vi "Test.vi"(11 "试验项目":T1(ring)) -> ()   [LabVIEW 2012]
uses:
  resultShow.vi
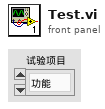
[diagram p1: front panel]
types:
  T1 = enum32{"功能", "输入输出特性", "电流特性", "传感器特性", "空载", "逆向空载", "振动", "7", "8", "9", "10", "11", "12", "13"}
  T2 = enum16{"selectdata", "selectsave", "selectlist", "selectshow"}
  T3 = cluster{"max":dbl, "min":dbl, "uripp":dbl, "average":dbl}
  T4 = cluster{"vaule":dbl, "vaule":dbl, "limitL":dbl, "limitH":dbl}
  T5 = typedef "svc_Spectrum Info.ctl" = cluster{"channel name":string, "description":string, "x-axis units":T6, "spectral info":cluster{"spectrum type":T7, "linear/dB":enum16{"linear", "dB"}, "window":u16, "window size":i32, "FFT size":i32}, "engineering units":T8, "custom label":string, "dB reference [EU]":dbl, "peak units":enum16{"rms", "peak", "peak-peak"}, "weighting filter":T9, "spectral density?":bool, "unit label":string, "spectrum skewed?":bool, "complimentary spectrum units":T10}
  T6 = typedef "svc_X-Axis Units.ctl" = u16
  T7 = typedef "svc_Spectrum Type.ctl" = enum16{"FFT Spectrum [complex]", "Amplitude [Magnitude]", "Power [Magnitude^2]", "Cross Spectrum [complex]", "Frequency Response [Complex]"}
  T8 = typedef "svc_Engineering Units Text Ring.ctl" = u16
  T9 = typedef "svc_Weighting Filter Text Ring.ctl" = u16
  T10 = typedef "svc_Complimentary Spectrum Units.ctl" = enum16{"none", "radians", "degrees", "cycles", "imaginary"}
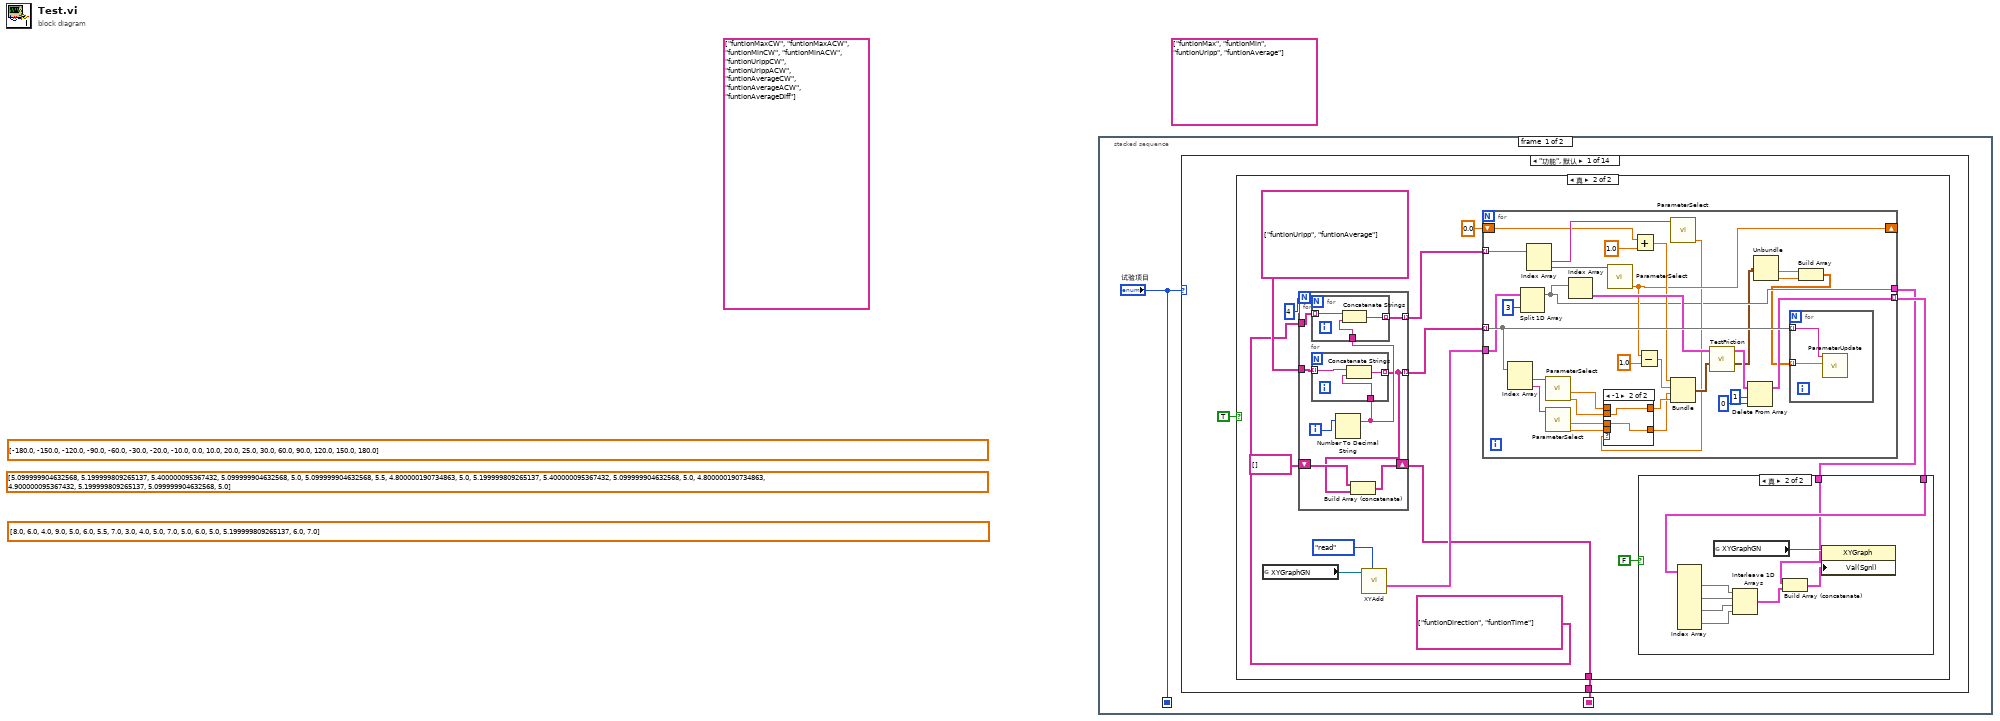
[diagram p0: block diagram]
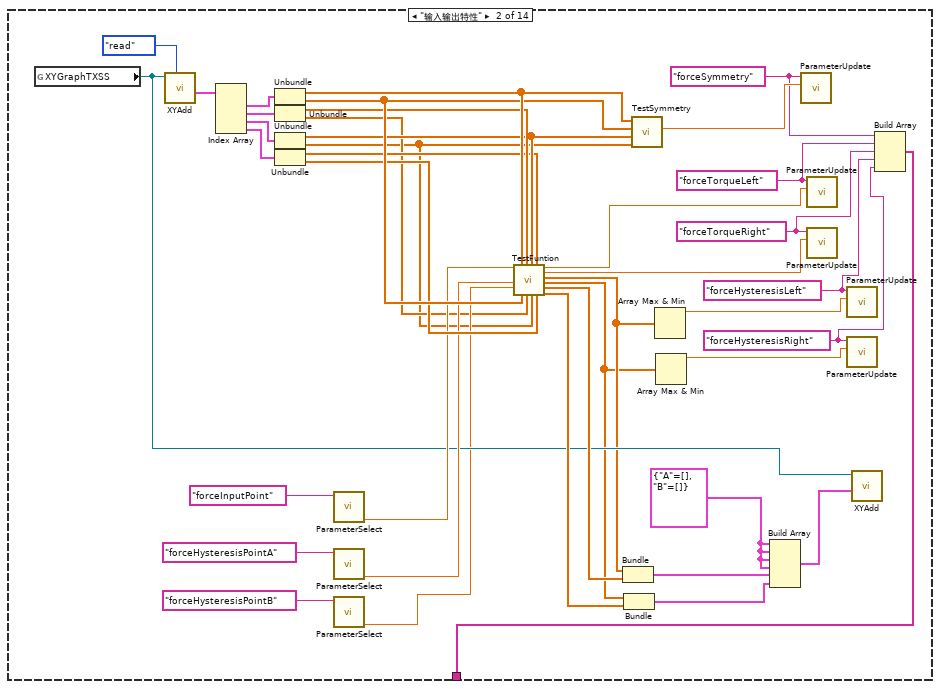
[diagram p5: hidden frame]
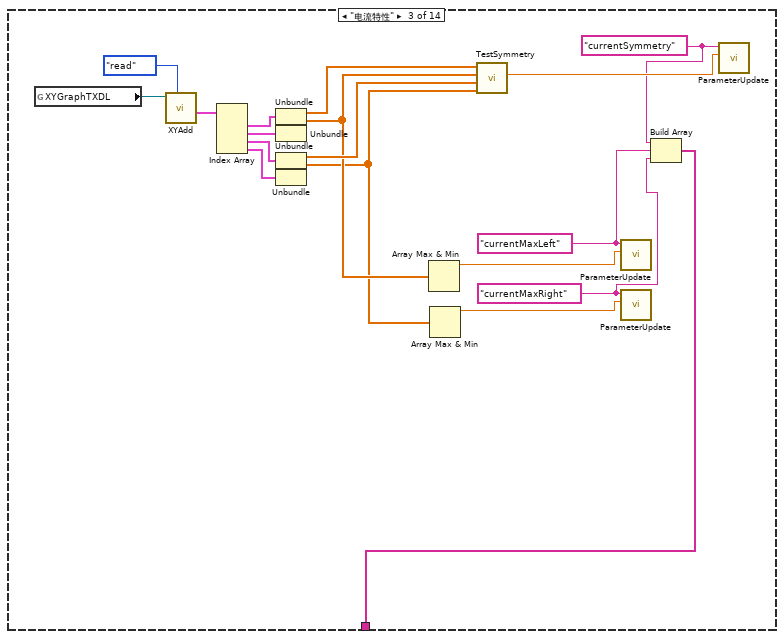
[diagram p6: hidden frame]
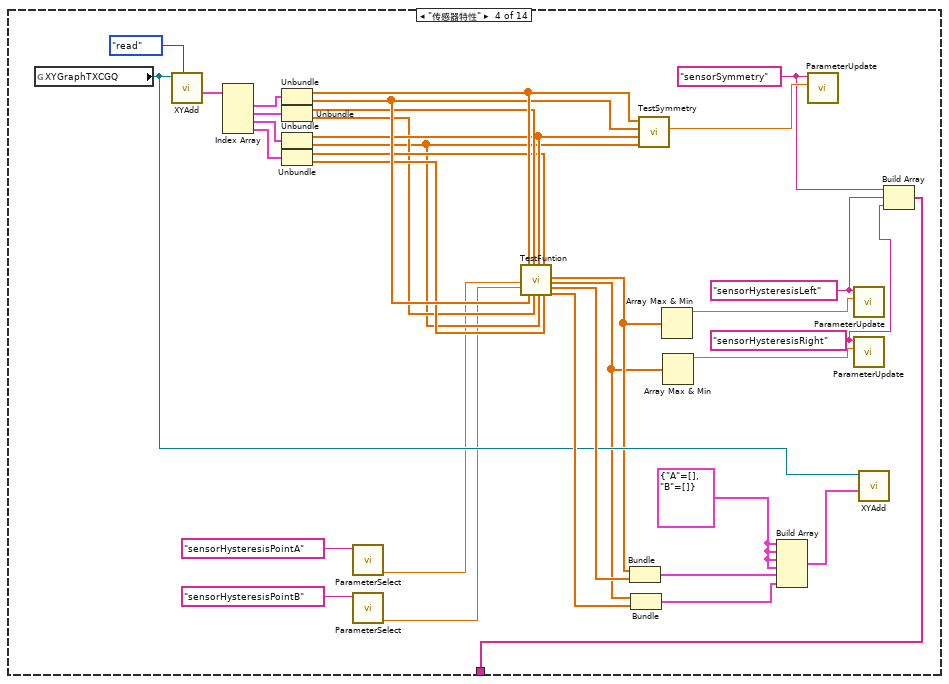
[diagram p7: hidden frame]
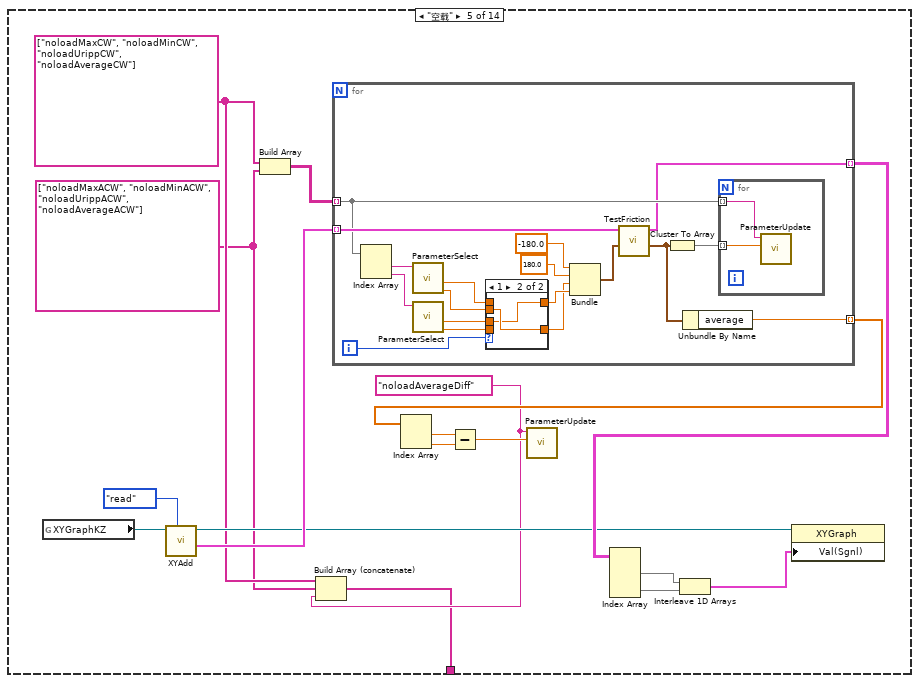
[diagram p8: hidden frame]
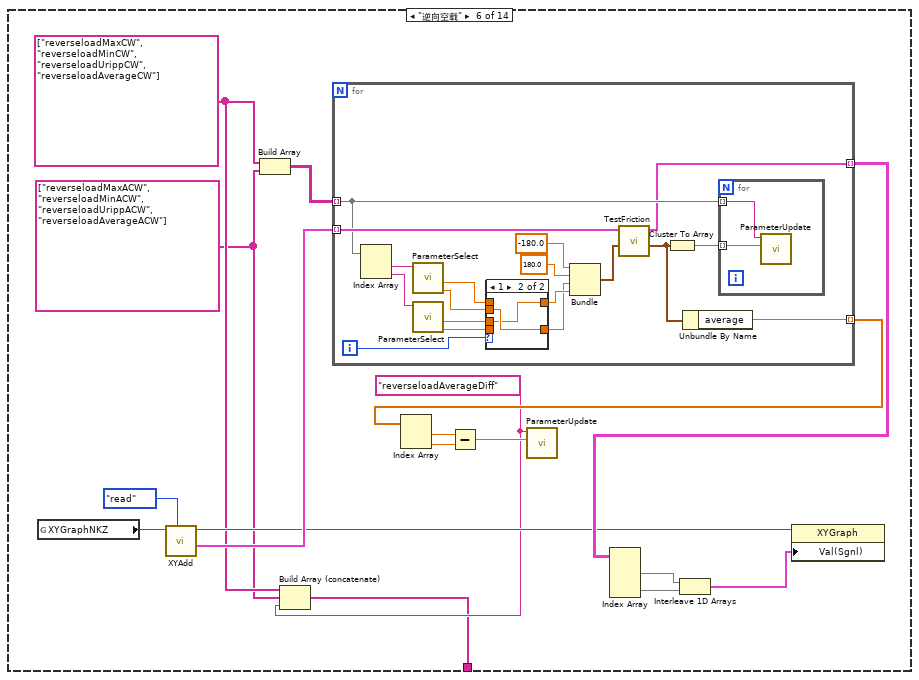
[diagram p10: hidden frame]
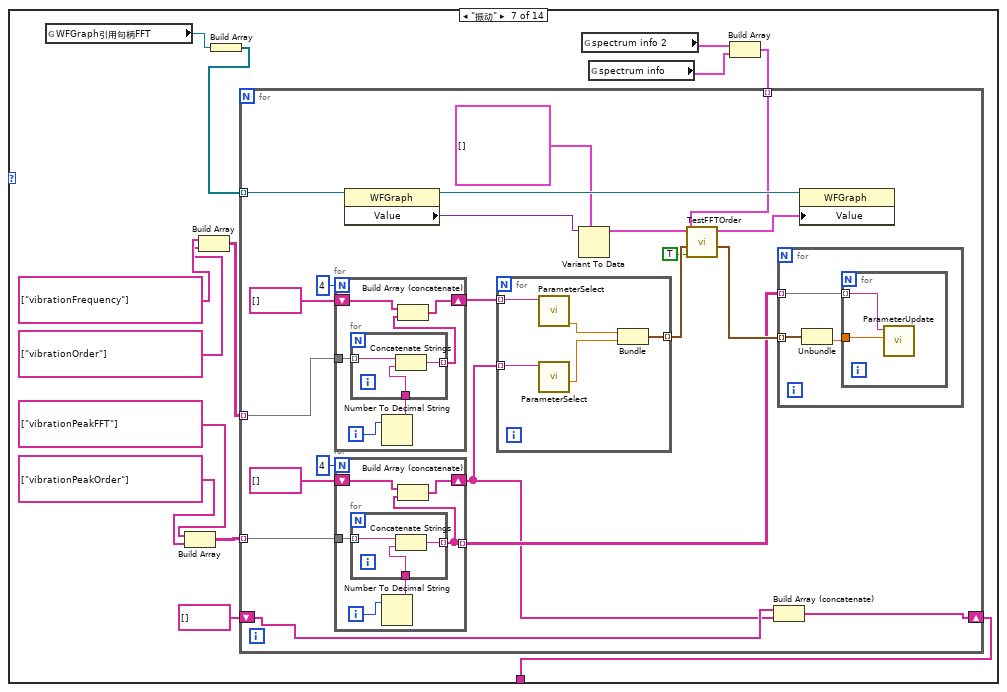
[diagram p12: hidden frame]
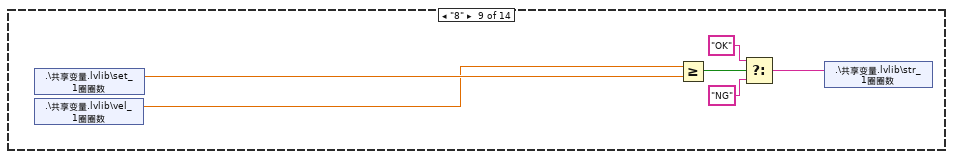
[diagram p14: hidden frame]
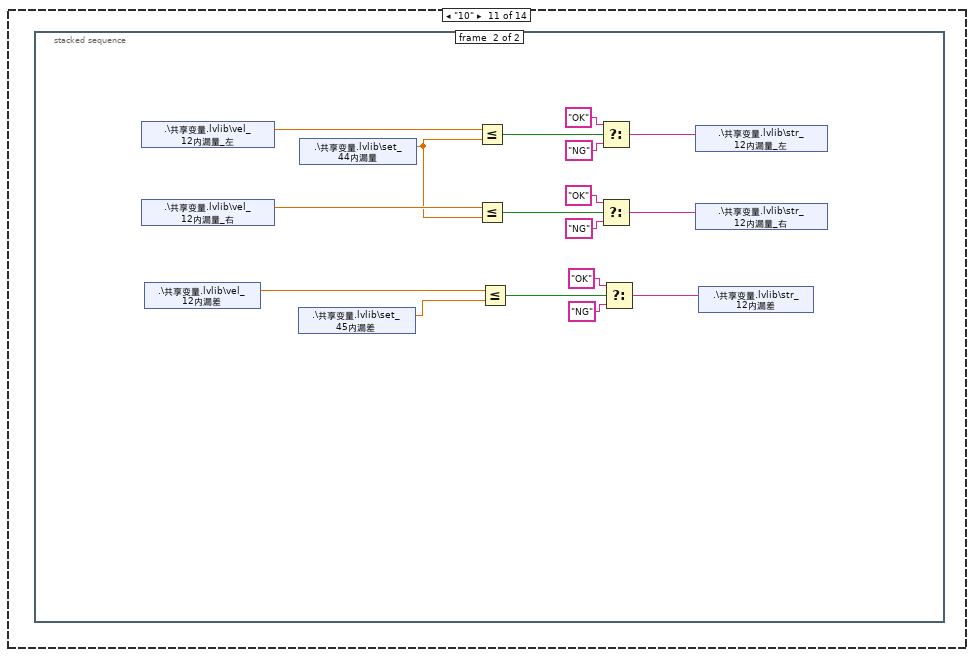
[diagram p17: hidden frame]
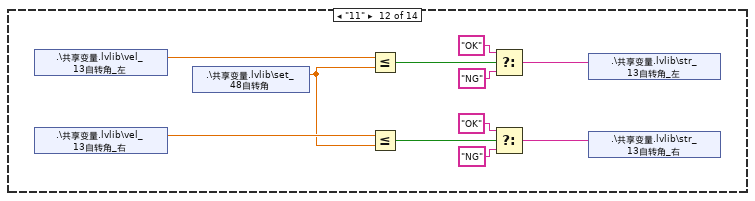
[diagram p19: hidden frame]
diagram:
  (unwired) string[] ["funtionMax", "funtionMin", "funtionUripp", "funtionAverage"] ("字符串[]")
  (unwired) string[] ["funtionMaxCW", "funtionMaxACW", "funtionMinCW", "funtionMinACW", "funtionUrippCW", "funtionUrippACW", "funtionAverageCW", "funtionAverageACW", "funtionAverageDiff"] ("字符串[]")
  (unwired) sgl[] [8.0, 6.0, 4.0, 9.0, 5.0, 6.0, 5.5, 7.0, 3.0, 4.0, 5.0, 7.0, 5.0, 6.0, 5.0, 5.2, 6.0, 7.0] ("Y")
  (unwired) sgl[] [5.1, 5.2, 5.4, 5.1, 5.0, 5.1, 5.5, 4.8, 5.0, 5.2, 5.4, 5.1, 5.0, 4.8, 4.9, 5.2, 5.1, 5.0] ("Y")
  (unwired) sgl[] [-180.0, -150.0, -120.0, -90.0, -60.0, -30.0, -20.0, -10.0, 0.0, 10.0, 20.0, 25.0, 30.0, 60.0, 90.0, 120.0, 150.0, 180.0] ("X")
  n1 = stacked-sequence {
    seq-local: [w2 _] -> [_ w359]
    seq-local: ["试验项目" _] -> [_ w358]
    frame #0 {
      n2 = case shown="\"功能\", 默认" "试验项目" {
        tunnel: [w4 w119 w120 w171 w172 w213 w254 _ _ _ _ _ _ _] -> w2
        frame "功能", Default {
          n3 = case shown="真" TRUE {
            tunnel: [_ w9] -> w4
            frame False {
            }
            frame True {
              n4 = global read "resultShow.vi" "XYGraphGN"() -> (w17:refnum<vi>)
              n5 = for {
                N: 4 -> [_]
                tunnel: string[] ["funtionUripp", "funtionAverage"] ("字符串[]") -> [w35]
                tunnel: [w29] -> w13 mode=indexing
                tunnel: [w32] -> w12 mode=indexing
                shift-right: [w31] -> w9
                shift-left: string[] [] -> [w30]
                tunnel: string[] ["funtionDirection", "funtionTime"] ("字符串[]") -> [w28]
                i -> [w34]
                n6 = Number To Decimal String(number=w34) -> (decimal integer string=w33:string)  [unwired: 1 in]
                n7 = for {
                  tunnel: w35 -> [w41] mode=indexing
                  tunnel: w33 -> [w40]
                  tunnel: [w39] -> w29 mode=indexing
                  n8 = Concatenate Strings(w41, w40) -> (w39:string)
                }
                n9 = for {
                  tunnel: w33 -> [w38]
                  tunnel: [w37] -> w32 mode=indexing
                  tunnel: w28 -> [w36] mode=indexing
                  n10 = Concatenate Strings(w36, w38) -> (w37:string)
                }
                n11 = Build Array (concatenate)(w30, w29) -> (w31:string[])
              }
              n12 = call "XYAdd.vi"("枚举"=enum16{"add", "read", "reset"}."read", "XYGraph"=w17) -> ("XYData"=w16:cluster{dbl[], dbl[]}[])  [unwired: 8 in, 1 out]
              n13 = for {
                tunnel: w16 -> [w48]
                tunnel: w13 -> [w73] mode=indexing
                tunnel: [w57] -> w7 mode=indexing
                tunnel: w12 -> [w63] mode=indexing
                shift-right: [w51] -> _
                shift-left: 0.0 ("limitL") -> [w54]
                tunnel: [w46] -> w6
                n14 = Index Array(array=w73) -> (element #1=w72:string, element #2=w71:string)  [unwired: 2 in]
                n15 = Split 1D Array(array=w48, index=3 ("索引")) -> (first subarray=w46:cluster{dbl[], dbl[]}[])  [unwired: 1 out]
                n16 = Index Array(array=w63) -> (element #1=w61:string, element #2=w62:string)  [unwired: 2 in]
                n17 = call "ParameterSelect.vi"("parameterName"=w72) -> ("limitL"=w65:dbl, "limitH"=w69:dbl)  [unwired: 5 in, 4 out]
                n18 = call "ParameterSelect.vi"("parameterName"=w71) -> ("limitL"=w67:dbl, "limitH"=w64:dbl)  [unwired: 5 in, 4 out]
                n19 = Index Array(array=w46) -> (element=w56:cluster{dbl[], dbl[]})  [unwired: 1 in]
                n20 = call "ParameterSelect.vi"("parameterName"=w62) -> ("limitL"=w51:dbl)  [unwired: 5 in, 5 out]
                n21 = Add(x=w54, y=1.0 ("vaule")) -> (x+y=w53:dbl)
                n22 = Subtract(x=w51, y=1.0 ("vaule")) -> (x-y=w50:dbl)
                n23 = call "ParameterSelect.vi"("parameterName"=w61) -> ("limitL"=w49:dbl)  [unwired: 5 in, 5 out]
                n24 = case shown="-1" w49 {
                  tunnel: w69 -> [w75 _]
                  tunnel: [w75 w76] -> w68
                  tunnel: w67 -> [w74 _]
                  tunnel: [w74 w77] -> w66
                  tunnel: w65 -> [_ w76]
                  tunnel: w64 -> [_ w77]
                  frame 1, Default {
                  }
                  frame -1 {
                  }
                }
                n25 = Bundle(w53, w50, "limitH"=w66, "limitL"=w68) -> (w70:cluster{dbl, dbl, "limitH":dbl, "limitL":dbl})  [unwired: 1 in]
                n26 = call "TestFriction.vi"("边界配置"=w70, "原始曲线"=w56) -> ("运算值"=w45:T3, "曲线数组"=w60:cluster{"X":dbl[], "Y":dbl[]}[])  [unwired: 8 in]
                n27 = Delete From Array(array=w60, length=1 ("长度"), index=0 ("索引")) -> (array with subset deleted=w57:cluster{"X":dbl[], "Y":dbl[]}[])  [unwired: 1 out]
                n28 = Unbundle(w45) -> ("uripp"=w44:dbl, "average"=w43:dbl)  [unwired: 2 out]
                n29 = Build Array(w44, w43) -> (w42:dbl[])
                n30 = for {
                  tunnel: w42 -> [w78] mode=indexing
                  tunnel: w73 -> [w79] mode=indexing
                  n31 = call "ParameterUpdate.vi"("vaule"=w78, "parameterName"=w79) -> ()  [unwired: 10 in]
                }
              }
              n32 = case shown="真" FALSE {
                tunnel: w7 -> [_ w25]
                tunnel: w6 -> [_ w19]
                frame False {
                }
                frame True {
                  n33 = Index Array(array=w25) -> (element #1=w27:cluster{"X":dbl[], "Y":dbl[]}[], element #2=w21:cluster{"X":dbl[], "Y":dbl[]}[], element #3=w22:cluster{"X":dbl[], "Y":dbl[]}[], element #4=w20:cluster{"X":dbl[], "Y":dbl[]}[])  [unwired: 8 in]
                  n34 = global read "resultShow.vi" "XYGraphGN"() -> (w26:refnum<vi>)
                  n35 = Interleave 1D Arrays(w27, w21, w22, w20) -> (w24:cluster{"X":dbl[], "Y":dbl[]}[])
                  n36 = Build Array (concatenate)(w19, w24) -> (w23:cluster{"X":dbl[], "Y":dbl[]}[])
                  n37 = property class="XYGraph"(reference=w26, "Val(Sgnl)"=w23) -> ()  [unwired: 1 in, 2 out]
                }
              }
            }
          }
        }
        frame "输入输出特性" {
          w93 = cluster{"A":dbl[], "B":dbl[]} {"A"=[], "B"=[]} ("元素")
          w86 = "forceHysteresisRight"
          w87 = "forceHysteresisLeft"
          w88 = "forceTorqueRight"
          w89 = "forceTorqueLeft"
          w90 = "forceSymmetry"
          n38 = global read "resultShow.vi" "XYGraphTXSS"() -> (w91:refnum<vi>)
          n39 = call "XYAdd.vi"("枚举"=enum16{"add", "read", "reset"}."read", "XYGraph"=w91) -> ("XYData"=w112:cluster{dbl[], dbl[]}[])  [unwired: 8 in, 1 out]
          n40 = Index Array(array=w112) -> (element #1=w113:cluster{dbl[], dbl[]}, element #2=w114:cluster{dbl[], dbl[]}, element #3=w115:cluster{dbl[], dbl[]}, element #4=w116:cluster{dbl[], dbl[]})  [unwired: 4 in]
          n41 = Unbundle(w113) -> (w110:dbl[], w109:dbl[])
          n42 = Unbundle(w114) -> (w108:dbl[], w83:dbl[])
          n43 = Unbundle(w115) -> (w107:dbl[], w82:dbl[])
          n44 = Unbundle(w116) -> (w106:dbl[], w105:dbl[])
          n45 = call "ParameterSelect.vi"("parameterName"="forceInputPoint") -> ("limitL"=w102:dbl)  [unwired: 5 in, 5 out]
          n46 = call "ParameterSelect.vi"("parameterName"="forceHysteresisPointA") -> ("limitL"=w101:dbl)  [unwired: 5 in, 5 out]
          n47 = call "ParameterSelect.vi"("parameterName"="forceHysteresisPointB") -> ("limitL"=w84:dbl)  [unwired: 5 in, 5 out]
          n48 = call "TestFuntion.vi"("定点输入设定"=w102, "滞后设定起始"=w101, "滞后设定结束"=w84, "x左升"=w110, "y左升"=w109, "x左回"=w108, "y左回"=w83, "x右升"=w107, "y右升"=w82, "x右回"=w106, "y右回"=w105) -> ("正输出定点"=w99:dbl, "逆输出定点"=w98:dbl, "正滞后x"=w81:dbl[], "逆滞后x"=w80:dbl[], "正滞后y"=w118:dbl[], "逆滞后y"=w117:dbl[])  [unwired: 3 in]
          n49 = Bundle("正滞后x"=w81, "正滞后y"=w118) -> (w94:cluster{"正滞后x":dbl[], "正滞后y":dbl[]})  [unwired: 1 in]
          n50 = Bundle("逆滞后x"=w80, "逆滞后y"=w117) -> (w92:cluster{"逆滞后x":dbl[], "逆滞后y":dbl[]})  [unwired: 1 in]
          n51 = call "TestSymmetry.vi"("Y右"=w82, "X右"=w107, "Y左"=w109, "X左"=w110) -> ("对称度"=w100:dbl)  [unwired: 7 in]
          n52 = Array Max & Min(array=w81) -> (max value=w97:dbl)  [unwired: 3 out]
          n53 = Array Max & Min(array=w80) -> (max value=w96:dbl)  [unwired: 3 out]
          n54 = Build Array(w93, w93, w93, w93, w94, w92) -> (w95:cluster{"逆滞后x":dbl[], "逆滞后y":dbl[]}[])
          n55 = call "ParameterUpdate.vi"("vaule"=w100, "parameterName"=w90) -> ()  [unwired: 10 in]
          n56 = call "ParameterUpdate.vi"("vaule"=w99, "parameterName"=w89) -> ()  [unwired: 10 in]
          n57 = call "ParameterUpdate.vi"("vaule"=w98, "parameterName"=w88) -> ()  [unwired: 10 in]
          n58 = call "ParameterUpdate.vi"("vaule"=w97, "parameterName"=w87) -> ()  [unwired: 10 in]
          n59 = call "ParameterUpdate.vi"("vaule"=w96, "parameterName"=w86) -> ()  [unwired: 10 in]
          n60 = call "XYAdd.vi"("数据"=w95, "XYGraph"=w91) -> ()  [unwired: 8 in, 2 out]
          n61 = Build Array(w90, w89, w88, w87, w86) -> (w119:string[])
        }
        frame "电流特性" {
          w124 = "currentMaxRight"
          w125 = "currentMaxLeft"
          w123 = "currentSymmetry"
          n62 = global read "resultShow.vi" "XYGraphTXDL"() -> (w131:refnum<vi>)
          n63 = call "XYAdd.vi"("枚举"=enum16{"add", "read", "reset"}."read", "XYGraph"=w131) -> ("XYData"=w133:cluster{dbl[], dbl[]}[])  [unwired: 8 in, 1 out]
          n64 = Index Array(array=w133) -> (element #1=w134:cluster{dbl[], dbl[]}, element #2=w135:cluster{dbl[], dbl[]}, element #3=w136:cluster{dbl[], dbl[]}, element #4=w137:cluster{dbl[], dbl[]})  [unwired: 4 in]
          n65 = Unbundle(w134) -> (w130:dbl[], w122:dbl[])
          n66 = Unbundle(w135) -> ()  [unwired: 2 out]
          n67 = Unbundle(w136) -> (w129:dbl[], w121:dbl[])
          n68 = Unbundle(w137) -> ()  [unwired: 2 out]
          n69 = Array Max & Min(array=w122) -> (max value=w127:dbl)  [unwired: 3 out]
          n70 = Array Max & Min(array=w121) -> (max value=w126:dbl)  [unwired: 3 out]
          n71 = call "TestSymmetry.vi"("Y右"=w121, "X右"=w129, "Y左"=w122, "X左"=w130) -> ("对称度"=w128:dbl)  [unwired: 7 in]
          n72 = call "ParameterUpdate.vi"("vaule"=w127, "parameterName"=w125) -> ()  [unwired: 10 in]
          n73 = call "ParameterUpdate.vi"("vaule"=w126, "parameterName"=w124) -> ()  [unwired: 10 in]
          n74 = Build Array(w123, w125, w124) -> (w120:string[])
          n75 = call "ParameterUpdate.vi"("vaule"=w128, "parameterName"=w123) -> ()  [unwired: 10 in]
        }
        frame "传感器特性" {
          w151 = cluster{"A":dbl[], "B":dbl[]} {"A"=[], "B"=[]} ("元素")
          w146 = "sensorHysteresisRight"
          w147 = "sensorHysteresisLeft"
          w148 = "sensorSymmetry"
          n76 = global read "resultShow.vi" "XYGraphTXCGQ"() -> (w149:refnum<vi>)
          n77 = call "XYAdd.vi"("枚举"=enum16{"add", "read", "reset"}."read", "XYGraph"=w149) -> ("XYData"=w164:cluster{dbl[], dbl[]}[])  [unwired: 8 in, 1 out]
          n78 = Index Array(array=w164) -> (element #1=w165:cluster{dbl[], dbl[]}, element #2=w166:cluster{dbl[], dbl[]}, element #3=w167:cluster{dbl[], dbl[]}, element #4=w168:cluster{dbl[], dbl[]})  [unwired: 4 in]
          n79 = Unbundle(w165) -> (w162:dbl[], w161:dbl[])
          n80 = Unbundle(w166) -> (w160:dbl[], w145:dbl[])
          n81 = Unbundle(w167) -> (w159:dbl[], w144:dbl[])
          n82 = Unbundle(w168) -> (w158:dbl[], w157:dbl[])
          n83 = call "ParameterSelect.vi"("parameterName"="sensorHysteresisPointA") -> ("limitL"=w141:dbl)  [unwired: 5 in, 5 out]
          n84 = call "ParameterSelect.vi"("parameterName"="sensorHysteresisPointB") -> ("limitL"=w140:dbl)  [unwired: 5 in, 5 out]
          n85 = call "TestFuntion.vi"("滞后设定起始"=w141, "滞后设定结束"=w140, "x左升"=w162, "y左升"=w161, "x左回"=w160, "y左回"=w145, "x右升"=w159, "y右升"=w144, "x右回"=w158, "y右回"=w157) -> ("正滞后x"=w139:dbl[], "逆滞后x"=w138:dbl[], "正滞后y"=w170:dbl[], "逆滞后y"=w169:dbl[])  [unwired: 4 in, 2 out]
          n86 = Bundle("正滞后x"=w139, "正滞后y"=w170) -> (w152:cluster{"正滞后x":dbl[], "正滞后y":dbl[]})  [unwired: 1 in]
          n87 = Bundle("逆滞后x"=w138, "逆滞后y"=w169) -> (w150:cluster{"逆滞后x":dbl[], "逆滞后y":dbl[]})  [unwired: 1 in]
          n88 = call "TestSymmetry.vi"("Y右"=w144, "X右"=w159, "Y左"=w161, "X左"=w162) -> ("对称度"=w156:dbl)  [unwired: 7 in]
          n89 = Array Max & Min(array=w139) -> (max value=w155:dbl)  [unwired: 3 out]
          n90 = Array Max & Min(array=w138) -> (max value=w154:dbl)  [unwired: 3 out]
          n91 = Build Array(w151, w151, w151, w151, w152, w150) -> (w153:cluster{"逆滞后x":dbl[], "逆滞后y":dbl[]}[])
          n92 = call "ParameterUpdate.vi"("vaule"=w156, "parameterName"=w148) -> ()  [unwired: 10 in]
          n93 = call "ParameterUpdate.vi"("vaule"=w155, "parameterName"=w147) -> ()  [unwired: 10 in]
          n94 = call "ParameterUpdate.vi"("vaule"=w154, "parameterName"=w146) -> ()  [unwired: 10 in]
          n95 = call "XYAdd.vi"("数据"=w153, "XYGraph"=w149) -> ()  [unwired: 8 in, 2 out]
          n96 = Build Array(w148, w147, w146) -> (w171:string[])
        }
        frame "空载" {
          w173 = "noloadAverageDiff"
          w174 = string[] ["noloadMaxACW", "noloadMinACW", "noloadUrippACW", "noloadAverageACW"] ("字符串[]")
          w175 = string[] ["noloadMaxCW", "noloadMinCW", "noloadUrippCW", "noloadAverageCW"] ("字符串[]")
          n97 = global read "resultShow.vi" "XYGraphKZ"() -> (w178:refnum<vi>)
          n98 = call "XYAdd.vi"("枚举"=enum16{"add", "read", "reset"}."read", "XYGraph"=w178) -> ("XYData"=w177:cluster{dbl[], dbl[]}[], "XYGraph 2"=w176:refnum<vi>)  [unwired: 8 in]
          n99 = Build Array(w175, w174) -> (w188:string[][])
          n100 = Build Array (concatenate)(w175, w174, w173) -> (w172:string[])
          n101 = for {
            tunnel: w177 -> [w206] mode=indexing
            tunnel: w188 -> [w202] mode=indexing
            tunnel: [w203] -> w187 mode=indexing
            tunnel: [w189] -> w180 mode=indexing
            i -> [w196]
            n102 = Index Array(array=w202) -> (element #1=w201:string, element #2=w200:string)  [unwired: 2 in]
            n103 = call "ParameterSelect.vi"("parameterName"=w201) -> ("limitL"=w191:dbl, "limitH"=w195:dbl)  [unwired: 5 in, 4 out]
            n104 = call "ParameterSelect.vi"("parameterName"=w200) -> ("limitL"=w193:dbl, "limitH"=w190:dbl)  [unwired: 5 in, 4 out]
            n105 = case shown="1" w196 {
              tunnel: w195 -> [w208 _]
              tunnel: [w208 w209] -> w194
              tunnel: w193 -> [w207 _]
              tunnel: [w207 w210] -> w192
              tunnel: w191 -> [_ w210]
              tunnel: w190 -> [_ w209]
              frame 0, Default {
              }
              frame 1 {
              }
            }
            n106 = Bundle("vaule"=-180.0, "vaule"=180.0, "limitL"=w192, "limitH"=w194) -> (w199:T4)  [unwired: 1 in]
            n107 = call "TestFriction.vi"("边界配置"=w199, "原始曲线"=w206) -> ("运算值"=w204:T3, "曲线数组"=w189:cluster{"X":dbl[], "Y":dbl[]}[])  [unwired: 8 in]
            n108 = Cluster To Array(cluster=w204) -> (array=w205:dbl[])
            n109 = Unbundle By Name(w204) -> ("average"=w203:dbl)
            n110 = for {
              tunnel: w205 -> [w211] mode=indexing
              tunnel: w202 -> [w212] mode=indexing
              n111 = call "ParameterUpdate.vi"("vaule"=w211, "parameterName"=w212) -> ()  [unwired: 10 in]
            }
          }
          n112 = Index Array(array=w187) -> (element #1=w185:dbl, element #2=w186:dbl)  [unwired: 2 in]
          n113 = Subtract(x=w185, y=w186) -> (x-y=w184:dbl)
          n114 = call "ParameterUpdate.vi"("vaule"=w184, "parameterName"=w173) -> ()  [unwired: 10 in]
          n115 = Index Array(array=w180) -> (element #1=w183:cluster{"X":dbl[], "Y":dbl[]}[], element #2=w182:cluster{"X":dbl[], "Y":dbl[]}[])  [unwired: 4 in]
          n116 = Interleave 1D Arrays(w183, w182) -> (w181:cluster{"X":dbl[], "Y":dbl[]}[])
          n117 = property class="XYGraph"(reference=w176, "Val(Sgnl)"=w181) -> ()  [unwired: 1 in, 2 out]
        }
        frame "逆向空载" {
          w214 = "reverseloadAverageDiff"
          w215 = string[] ["reverseloadMaxACW", "reverseloadMinACW", "reverseloadUrippACW", "reverseloadAverageACW"] ("字符串[]")
          w216 = string[] ["reverseloadMaxCW", "reverseloadMinCW", "reverseloadUrippCW", "reverseloadAverageCW"] ("字符串[]")
          n118 = global read "resultShow.vi" "XYGraphNKZ"() -> (w219:refnum<vi>)
          n119 = call "XYAdd.vi"("枚举"=enum16{"add", "read", "reset"}."read", "XYGraph"=w219) -> ("XYData"=w218:cluster{dbl[], dbl[]}[], "XYGraph 2"=w217:refnum<vi>)  [unwired: 8 in]
          n120 = Build Array(w216, w215) -> (w229:string[][])
          n121 = Build Array (concatenate)(w216, w215, w214) -> (w213:string[])
          n122 = for {
            tunnel: w218 -> [w247] mode=indexing
            tunnel: w229 -> [w243] mode=indexing
            tunnel: [w244] -> w228 mode=indexing
            tunnel: [w230] -> w221 mode=indexing
            i -> [w237]
            n123 = Index Array(array=w243) -> (element #1=w242:string, element #2=w241:string)  [unwired: 2 in]
            n124 = call "ParameterSelect.vi"("parameterName"=w242) -> ("limitL"=w232:dbl, "limitH"=w236:dbl)  [unwired: 5 in, 4 out]
            n125 = call "ParameterSelect.vi"("parameterName"=w241) -> ("limitL"=w234:dbl, "limitH"=w231:dbl)  [unwired: 5 in, 4 out]
            n126 = case shown="1" w237 {
              tunnel: w236 -> [w249 _]
              tunnel: [w249 w250] -> w235
              tunnel: w234 -> [w248 _]
              tunnel: [w248 w251] -> w233
              tunnel: w232 -> [_ w251]
              tunnel: w231 -> [_ w250]
              frame 0, Default {
              }
              frame 1 {
              }
            }
            n127 = Bundle("vaule"=-180.0, "vaule"=180.0, "limitL"=w233, "limitH"=w235) -> (w240:T4)  [unwired: 1 in]
            n128 = call "TestFriction.vi"("边界配置"=w240, "原始曲线"=w247) -> ("运算值"=w245:T3, "曲线数组"=w230:cluster{"X":dbl[], "Y":dbl[]}[])  [unwired: 8 in]
            n129 = Cluster To Array(cluster=w245) -> (array=w246:dbl[])
            n130 = Unbundle By Name(w245) -> ("average"=w244:dbl)
            n131 = for {
              tunnel: w246 -> [w252] mode=indexing
              tunnel: w243 -> [w253] mode=indexing
              n132 = call "ParameterUpdate.vi"("vaule"=w252, "parameterName"=w253) -> ()  [unwired: 10 in]
            }
          }
          n133 = Index Array(array=w228) -> (element #1=w226:dbl, element #2=w227:dbl)  [unwired: 2 in]
          n134 = Subtract(x=w226, y=w227) -> (x-y=w225:dbl)
          n135 = call "ParameterUpdate.vi"("vaule"=w225, "parameterName"=w214) -> ()  [unwired: 10 in]
          n136 = Index Array(array=w221) -> (element #1=w224:cluster{"X":dbl[], "Y":dbl[]}[], element #2=w223:cluster{"X":dbl[], "Y":dbl[]}[])  [unwired: 4 in]
          n137 = Interleave 1D Arrays(w224, w223) -> (w222:cluster{"X":dbl[], "Y":dbl[]}[])
          n138 = property class="XYGraph"(reference=w217, "Val(Sgnl)"=w222) -> ()  [unwired: 1 in, 2 out]
        }
        frame "振动" {
          n139 = global read "resultShow.vi" "WFGraph引用句柄FFT"() -> (w266:refnum<vi>)
          n140 = Build Array(string[] ["vibrationPeakFFT"] ("字符串[]"), string[] ["vibrationPeakOrder"] ("字符串[]")) -> (w259:string[][])
          n141 = Build Array(string[] ["vibrationFrequency"] ("字符串[]"), string[] ["vibrationOrder"] ("字符串[]")) -> (w262:string[][])
          n142 = Build Array(w266) -> (w265:refnum<vi>[])
          n143 = global read "resultShow.vi" "spectrum info 2"() -> (w258:T5)
          n144 = global read "resultShow.vi" "spectrum info"() -> (w257:T5)
          n145 = Build Array(w258, w257) -> (w256:T5[])
          n146 = for {
            tunnel: w265 -> [w274] mode=indexing
            tunnel: w262 -> [w273] mode=indexing
            tunnel: w259 -> [w272] mode=indexing
            tunnel: w256 -> [w271] mode=indexing
            shift-right: [w270] -> w254
            shift-left: string[] [] -> [w269]
            n147 = for {
              N: 4 -> [_]
              tunnel: w273 -> [w312]
              shift-right: [w309] -> w279
              shift-left: string[] [] -> [w308]
              i -> [w311]
              n148 = Number To Decimal String(number=w311) -> (decimal integer string=w310:string)  [unwired: 1 in]
              n149 = for {
                tunnel: w312 -> [w315] mode=indexing
                tunnel: w310 -> [w314]
                tunnel: [w313] -> w307 mode=indexing
                n150 = Concatenate Strings(w315, w314) -> (w313:string)
              }
              n151 = Build Array (concatenate)(w308, w307) -> (w309:string[])
            }
            n152 = for {
              N: 4 -> [_]
              tunnel: w272 -> [w298]
              shift-right: [w295] -> w268
              shift-left: string[] [] -> [w294]
              tunnel: [w293] -> w275 mode=indexing
              i -> [w297]
              n153 = Number To Decimal String(number=w297) -> (decimal integer string=w296:string)  [unwired: 1 in]
              n154 = for {
                tunnel: w298 -> [w301] mode=indexing
                tunnel: w296 -> [w300]
                tunnel: [w299] -> w293 mode=indexing
                n155 = Concatenate Strings(w301, w300) -> (w299:string)
              }
              n156 = Build Array (concatenate)(w294, w293) -> (w295:string[])
            }
            n157 = property class="WFGraph"(reference=w274) -> (reference out=w287:refnum<vi>, "Value"=w286:variant)  [unwired: 1 in, 1 out]
            n158 = for {
              tunnel: w279 -> [w306] mode=indexing
              tunnel: [w303] -> w280 mode=indexing
              tunnel: w268 -> [w302] mode=indexing
              n159 = call "ParameterSelect.vi"("parameterName"=w306) -> ("limitL"=w305:dbl)  [unwired: 5 in, 5 out]
              n160 = call "ParameterSelect.vi"("parameterName"=w302) -> ("limitH"=w304:dbl)  [unwired: 5 in, 5 out]
              n161 = Bundle("limitL"=w305, "limitH"=w304) -> (w303:cluster{"limitL":dbl, "limitH":dbl})  [unwired: 1 in]
            }
            n162 = Variant To Data(type=cluster{"x0":dbl, "dx":dbl, "Y":dbl[]}[] [] ("FFT 2"), Variant=w286) -> (data=w284:cluster{"x0":dbl, "dx":dbl, "Y":dbl[]}[])  [unwired: 1 in, 1 out]
            n163 = call "TestFFTOrder.vi"("布尔"=TRUE, 9:w280, "spectrum info 2"=w271, "FFT 5"=w284) -> ("数组"=w276:cluster{"freq.":dbl, "dB":dbl}[], "FFT 2"=w283:cluster{"x0":dbl, "dx":dbl, "Y":dbl[]}[])  [unwired: 6 in]
            n164 = Build Array (concatenate)(w269, w268) -> (w270:string[])
            n165 = for {
              tunnel: w275 -> [w290] mode=indexing
              tunnel: w276 -> [w289] mode=indexing
              n166 = Unbundle(w289) -> ("dB"=w288:dbl)  [unwired: 1 out]
              n167 = for {
                tunnel: w288 -> [w291]
                tunnel: w290 -> [w292] mode=indexing
                n168 = call "ParameterUpdate.vi"("vaule"=w291, "parameterName"=w292) -> ()  [unwired: 10 in]
              }
            }
            n169 = property class="WFGraph"(reference=w287, "Value"=w283) -> ()  [unwired: 1 in, 2 out]
          }
        }
        frame "7" {
        }
        frame "8" {
          n170 = shared-variable ".\\共享变量.lvlib\\set_1圈圈数"() -> (w318:sgl)  [unwired: 1 in, 1 out]
          n171 = shared-variable ".\\共享变量.lvlib\\vel_1圈圈数"() -> (w317:sgl)  [unwired: 1 in, 1 out]
          n172 = Greater Or Equal?(x=w317, y=w318) -> (x >= y?=w319:bool)
          n173 = Select(t="OK" ("str_1圈圈数"), s=w319, f="NG" ("str_1圈圈数")) -> (s? t:f=w316:string)
          n174 = shared-variable ".\\共享变量.lvlib\\str_1圈圈数"(w316) -> ()  [unwired: 1 in, 1 out]
        }
        frame "9" {
          n175 = stacked-sequence {
            frame #0 {
            }
            frame #1 {
            }
          }
        }
        frame "10" {
          n176 = stacked-sequence {
            frame #0 {
            }
            frame #1 {
              n177 = shared-variable ".\\共享变量.lvlib\\vel_12内漏量_左"() -> (w334:sgl)  [unwired: 1 in, 1 out]
              n178 = shared-variable ".\\共享变量.lvlib\\vel_12内漏量_右"() -> (w333:sgl)  [unwired: 1 in, 1 out]
              n179 = shared-variable ".\\共享变量.lvlib\\vel_12内漏差"() -> (w323:sgl)  [unwired: 1 in, 1 out]
              n180 = shared-variable ".\\共享变量.lvlib\\set_45内漏差"() -> (w322:sgl)  [unwired: 1 in, 1 out]
              n181 = shared-variable ".\\共享变量.lvlib\\set_44内漏量"() -> (w328:sgl)  [unwired: 1 in, 1 out]
              n182 = Less Or Equal?(x=w334, y=w328) -> (x <= y?=w336:bool)
              n183 = Less Or Equal?(x=w333, y=w328) -> (x <= y?=w331:bool)
              n184 = Less Or Equal?(x=w323, y=w322) -> (x <= y?=w325:bool)
              n185 = Select(t="OK" ("str_1圈圈数"), s=w336, f="NG" ("str_1圈圈数")) -> (s? t:f=w335:string)
              n186 = Select(t="OK" ("str_1圈圈数"), s=w331, f="NG" ("str_1圈圈数")) -> (s? t:f=w332:string)
              n187 = Select(t="OK" ("str_1圈圈数"), s=w325, f="NG" ("str_1圈圈数")) -> (s? t:f=w324:string)
              n188 = shared-variable ".\\共享变量.lvlib\\str_12内漏量_左"(w335) -> ()  [unwired: 1 in, 1 out]
              n189 = shared-variable ".\\共享变量.lvlib\\str_12内漏量_右"(w332) -> ()  [unwired: 1 in, 1 out]
              n190 = shared-variable ".\\共享变量.lvlib\\str_12内漏差"(w324) -> ()  [unwired: 1 in, 1 out]
            }
          }
        }
        frame "11" {
          n191 = shared-variable ".\\共享变量.lvlib\\vel_13自转角_左"() -> (w345:sgl)  [unwired: 1 in, 1 out]
          n192 = shared-variable ".\\共享变量.lvlib\\vel_13自转角_右"() -> (w344:sgl)  [unwired: 1 in, 1 out]
          n193 = shared-variable ".\\共享变量.lvlib\\set_48自转角"() -> (w339:sgl)  [unwired: 1 in, 1 out]
          n194 = Less Or Equal?(x=w345, y=w339) -> (x <= y?=w347:bool)
          n195 = Less Or Equal?(x=w344, y=w339) -> (x <= y?=w342:bool)
          n196 = Select(t="OK" ("str_1圈圈数"), s=w347, f="NG" ("str_1圈圈数")) -> (s? t:f=w346:string)
          n197 = Select(t="OK" ("str_1圈圈数"), s=w342, f="NG" ("str_1圈圈数")) -> (s? t:f=w343:string)
          n198 = shared-variable ".\\共享变量.lvlib\\str_13自转角_左"(w346) -> ()  [unwired: 1 in, 1 out]
          n199 = shared-variable ".\\共享变量.lvlib\\str_13自转角_右"(w343) -> ()  [unwired: 1 in, 1 out]
        }
        frame "12" {
        }
        frame "13" {
          n200 = shared-variable ".\\共享变量.lvlib\\vel_14压损失"() -> (w351:sgl)  [unwired: 1 in, 1 out]
          n201 = shared-variable ".\\共享变量.lvlib\\set_53压损失"() -> (w350:sgl)  [unwired: 1 in, 1 out]
          n202 = Less Or Equal?(x=w351, y=w350) -> (x <= y?=w353:bool)
          n203 = Select(t="OK" ("str_1圈圈数"), s=w353, f="NG" ("str_1圈圈数")) -> (s? t:f=w352:string)
          n204 = shared-variable ".\\共享变量.lvlib\\str_14压损失"(w352) -> ()  [unwired: 1 in, 1 out]
        }
      }
    }
    frame #1 {
      n205 = call "ParameterSelect.vi"("模式"=T2."selectshow") -> ("dataOutAll"=w357:string[][])  [unwired: 5 in, 5 out]
      n206 = for {
        tunnel: w357 -> [w365] mode=indexing
        tunnel: [w364] -> w356 mode=indexing
        n207 = for {
          tunnel: w365 -> [w369] mode=indexing
          tunnel: [w375] -> w364 mode=indexing
          i -> [w374]
          n208 = Empty String/Path?(string/path=w369) -> (empty?=w368:bool)
          n209 = Greater?(x=w374, y=0) -> (0:w371:bool)
          n210 = Less?(x=w374, y=4) -> (x < y?=w370:bool)
          n211 = Not(x=w368) -> (.not. x?=w367:bool)
          n212 = Compound Arithmetic op=AND(w367, w371, w370) -> (w366:bool)
          n213 = case shown="真" w366 {
            tunnel: [w376 w377] -> w375
            tunnel: w369 -> [w376 w382]
            frame False {
            }
            frame True {
              n214 = Fract/Exp String To Number(string=w382, default (0 dbl)=nan ("默认(0 DBL)")) -> (number=w383:dbl)  [unwired: 2 in, 1 out]
              n215 = Number To Fractional String(number=w383, precision (6)=i16 2 ("精度(6)")) -> (F-format string=w380:string)  [unwired: 2 in]
              n216 = Search and Replace String(input string=w380, search string=".00" ("搜索字符串"), replace string="" ("替换字符串(\"\")")) -> (result string=w377:string)  [unwired: 5 in, 3 out]
            }
          }
        }
      }
      n217 = global read "resultShow.vi" "TblRefFormMainShow"() -> (w362:refnum<vi>)
      n218 = global read "resultShow.vi" "LED"() -> (w361:refnum<vi>[])
      n219 = Index Array(array=w361, index=w358) -> (element=w360:refnum<vi>)
      n220 = property class="Tbl"(reference=w362, "Val(Sgnl)"=w356) -> ()  [unwired: 1 in, 2 out]
      n221 = for {
        tunnel: w359 -> [w389] mode=indexing
        tunnel: w360 -> [w386]
        stop <- w388 stop-if-true
        n222 = call "ParameterSelect.vi"("parameterName"=w389) -> ("result"=w385:string)  [unwired: 5 in, 5 out]
        n223 = Equal?(x=w385, y="×" ("元素")) -> (x = y?=w388:bool)
        n224 = call "Colour.vi"("result"=w385, "colourRef"=w386) -> ()  [unwired: 9 in, 1 out]
      }
    }
  }
